vi "Start New Test.vi"(8 "error in (no error)":errorcluster, 11 "Test Information":T2={"APU Part Number:"="", "Model:"="", "Serial Number:"="", "Customer:"="", "Work Order:"="", "Pre or Post SB"="", "Run Count"=0, "APU Selected"="<Select>"} {"Run Count" min=0 step=1}) -> (0 "error out":errorcluster)   [LabVIEW 2018, in "File IO.lvlib"]
doc: "This subVI enqueues the named action in to the communications queue along with the input data."
uses:
  File IO.lvlib
  Controller (Host)/Public Controls/Test Information.ctl
  Controller (Host)/Public VIs/PreorPostSB.ctl
  Controller (Host)/Public Controls/APU Select.ctl
  Private Controls/Module Action.ctl
  Private Controls/Module Data.ctl
  Controller (Host)/Controller (Host).lvlib
panel:
  in  "Action":T1=enum."Start New Test"
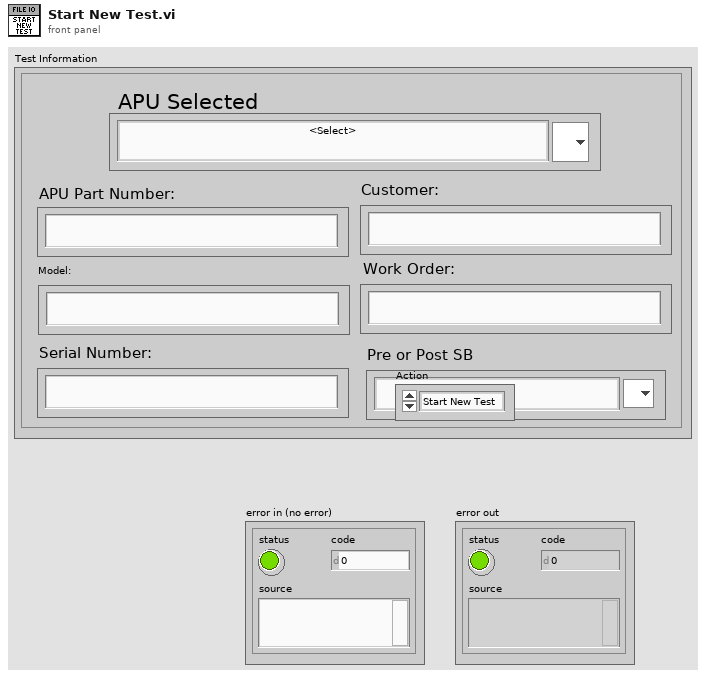
[diagram p1: front panel]
types:
  T1 = typedef "File IO.lvlib/Module Action.ctl" = enum8{"Timeout", "OpenReport", "Continue Test", "Init", "Error", "Exit", "Save Accel Data", "Set Recording State", "Log APU RunTime", "Start New Test", "Create New Reports", "Write to System Log", "Save Variables", "Load APU Setup File", "Increment Run Count", "Write To Report"}
  T2 = typedef "Controller (Host).lvlib/Test Information.ctl" = cluster{"APU Part Number:":string, "Model:":string, "Serial Number:":string, "Customer:":string, "Work Order:":string, "Pre or Post SB":T3, "Run Count":i32, "APU Selected":T4}
  T3 = typedef "Controller (Host).lvlib/PreorPostSB.ctl" = string
  T4 = typedef "Controller (Host).lvlib/APU Select.ctl" = string
  T5 = typedef "File IO.lvlib/Module Data.ctl" = cluster{"Data":variant, "Action":T1}
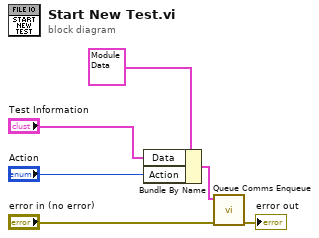
[diagram p0: block diagram]
diagram:
  n1 = Bundle By Name(cluster=T5 {"Data"=variant, "Action"=enum."Init"} ("element"), "Data"="Test Information", "Action"="Action") -> (w5:T5)
  n2 = call "Queue Comms Enqueue.vi"("error in (no error)"="error in (no error)", "element"=w5) -> ("error out"=→"error out":errorcluster)  [unwired: 9 in]
